vi "Outputs.vi"(8 "error in (no error)":errorcluster, 11 "State in":T1={"State"=enum."Idle", "Start Time"=timestamp(0 s since 1904-01-01), "Configuration"={"Cycle Period"=0.0, "PID 2 Parameters"={"Input Device"=enum."4-20mA", "Output Device"=enum."Default", "Setpoint"=0.0, "PID gains"={"proportional gain (Kc)"=0.0, "integral time (Ti, min)"=0.0, "derivative time (Td, min)"=100.0}, "output range"={"output low"=0.0, "output high"=1.0}}, "Manual Entry"=0.0, "Auto?"=TRUE, "4-20mA Input Settings"={"Input Channel "=0}, "4-20mA Out Settings"={"Output DAQ Task"=""}, "Input Channel Tag Name "=""}, "Current Time"=timestamp(0 s since 1904-01-01), "PID 1 Parameters"={"Setpoint"=0.0, "PID gains"={"proportional gain (Kc)"=1.0, "integral time (Ti, min)"=0.01, "derivative time (Td, min)"=0.0}}, "First Iteration"=FALSE, "Data"={"4-20mA Input"=0.0, "PID 2 Process Variable"=0.0, "PID 2 Output"=0.0, "4-20mA Output"=0.0}, "Process Name"="", "Pump On?"=enum."Off", "Input Error"=FALSE, "Output Error"=FALSE, "Log Started"=FALSE, "Current Setpoint"=0.0} {"Configuration"."PID 2 Parameters"."output range"."output low" format="%.2f"; "Configuration"."PID 2 Parameters"."output range"."output high" min=0.0 max=100.0 format="%.2f"; "Configuration"."PID 2 Parameters"."PID gains"."derivative time (Td, min)" format="%.3f"; "Configuration"."PID 2 Parameters"."PID gains"."integral time (Ti, min)" format="%.3f"; "Configuration"."PID 2 Parameters"."PID gains"."proportional gain (Kc)" format="%.3f"; "PID 1 Parameters"."PID gains"."derivative time (Td, min)" format="%.3f"; "PID 1 Parameters"."PID gains"."integral time (Ti, min)" format="%.3f"; "PID 1 Parameters"."PID gains"."proportional gain (Kc)" format="%.3f"}) -> (0 "error out":errorcluster, 3 "State out":T1={"State"=enum."Idle", "Start Time"=timestamp(0 s since 1904-01-01), "Configuration"={"Cycle Period"=0.0, "PID 2 Parameters"={"Input Device"=enum."4-20mA", "Output Device"=enum."Default", "Setpoint"=0.0, "PID gains"={"proportional gain (Kc)"=0.0, "integral time (Ti, min)"=0.0, "derivative time (Td, min)"=100.0}, "output range"={"output low"=0.0, "output high"=1.0}}, "Manual Entry"=0.0, "Auto?"=TRUE, "4-20mA Input Settings"={"Input Channel "=0}, "4-20mA Out Settings"={"Output DAQ Task"=""}, "Input Channel Tag Name "=""}, "Current Time"=timestamp(0 s since 1904-01-01), "PID 1 Parameters"={"Setpoint"=0.0, "PID gains"={"proportional gain (Kc)"=1.0, "integral time (Ti, min)"=0.01, "derivative time (Td, min)"=0.0}}, "First Iteration"=FALSE, "Data"={"4-20mA Input"=0.0, "PID 2 Process Variable"=0.0, "PID 2 Output"=0.0, "4-20mA Output"=0.0}, "Process Name"="", "Pump On?"=enum."Off", "Input Error"=FALSE, "Output Error"=FALSE, "Log Started"=FALSE, "Current Setpoint"=0.0} {"Configuration"."PID 2 Parameters"."output range"."output low" format="%.2f"; "Configuration"."PID 2 Parameters"."output range"."output high" min=0.0 max=100.0 format="%.2f"; "Configuration"."PID 2 Parameters"."PID gains"."derivative time (Td, min)" format="%.3f"; "Configuration"."PID 2 Parameters"."PID gains"."integral time (Ti, min)" format="%.3f"; "Configuration"."PID 2 Parameters"."PID gains"."proportional gain (Kc)" format="%.3f"; "PID 1 Parameters"."PID gains"."derivative time (Td, min)" format="%.3f"; "PID 1 Parameters"."PID gains"."integral time (Ti, min)" format="%.3f"; "PID 1 Parameters"."PID gains"."proportional gain (Kc)" format="%.3f"})   [LabVIEW 2018, in "4-20mA Module.lvlib" / "4-20mA Module Engine.lvlib"]
uses:
  4-20mA Module Engine.lvlib
  State Cluster.ctl
  State Enum.ctl
  Pressure Transmitter/Pressure Transmitter Device Settings.ctl
  Pressure Reg Module/Pressure Regulator Device Settings.ctl
  Measure Instrument/PID 1 Parameters Cluster.ctl
  Tag VIs/Tag FGV Operation Enum.ctl
  Shared Variables/Dynamic Shared Variables.lvlib
  Pressure Reg Module/Pressure Regulator Library.lvlib
  Flow Regulator/Pressure Reg Module/Flow Regulator Library.lvlib
  Pressure Transmitter/Pressure Transmitter Library.lvlib
panel:
  # "Instrument Settings"
  # "Instrument Settings"
  # "Instrument Settings"
  # "Instrument Settings"
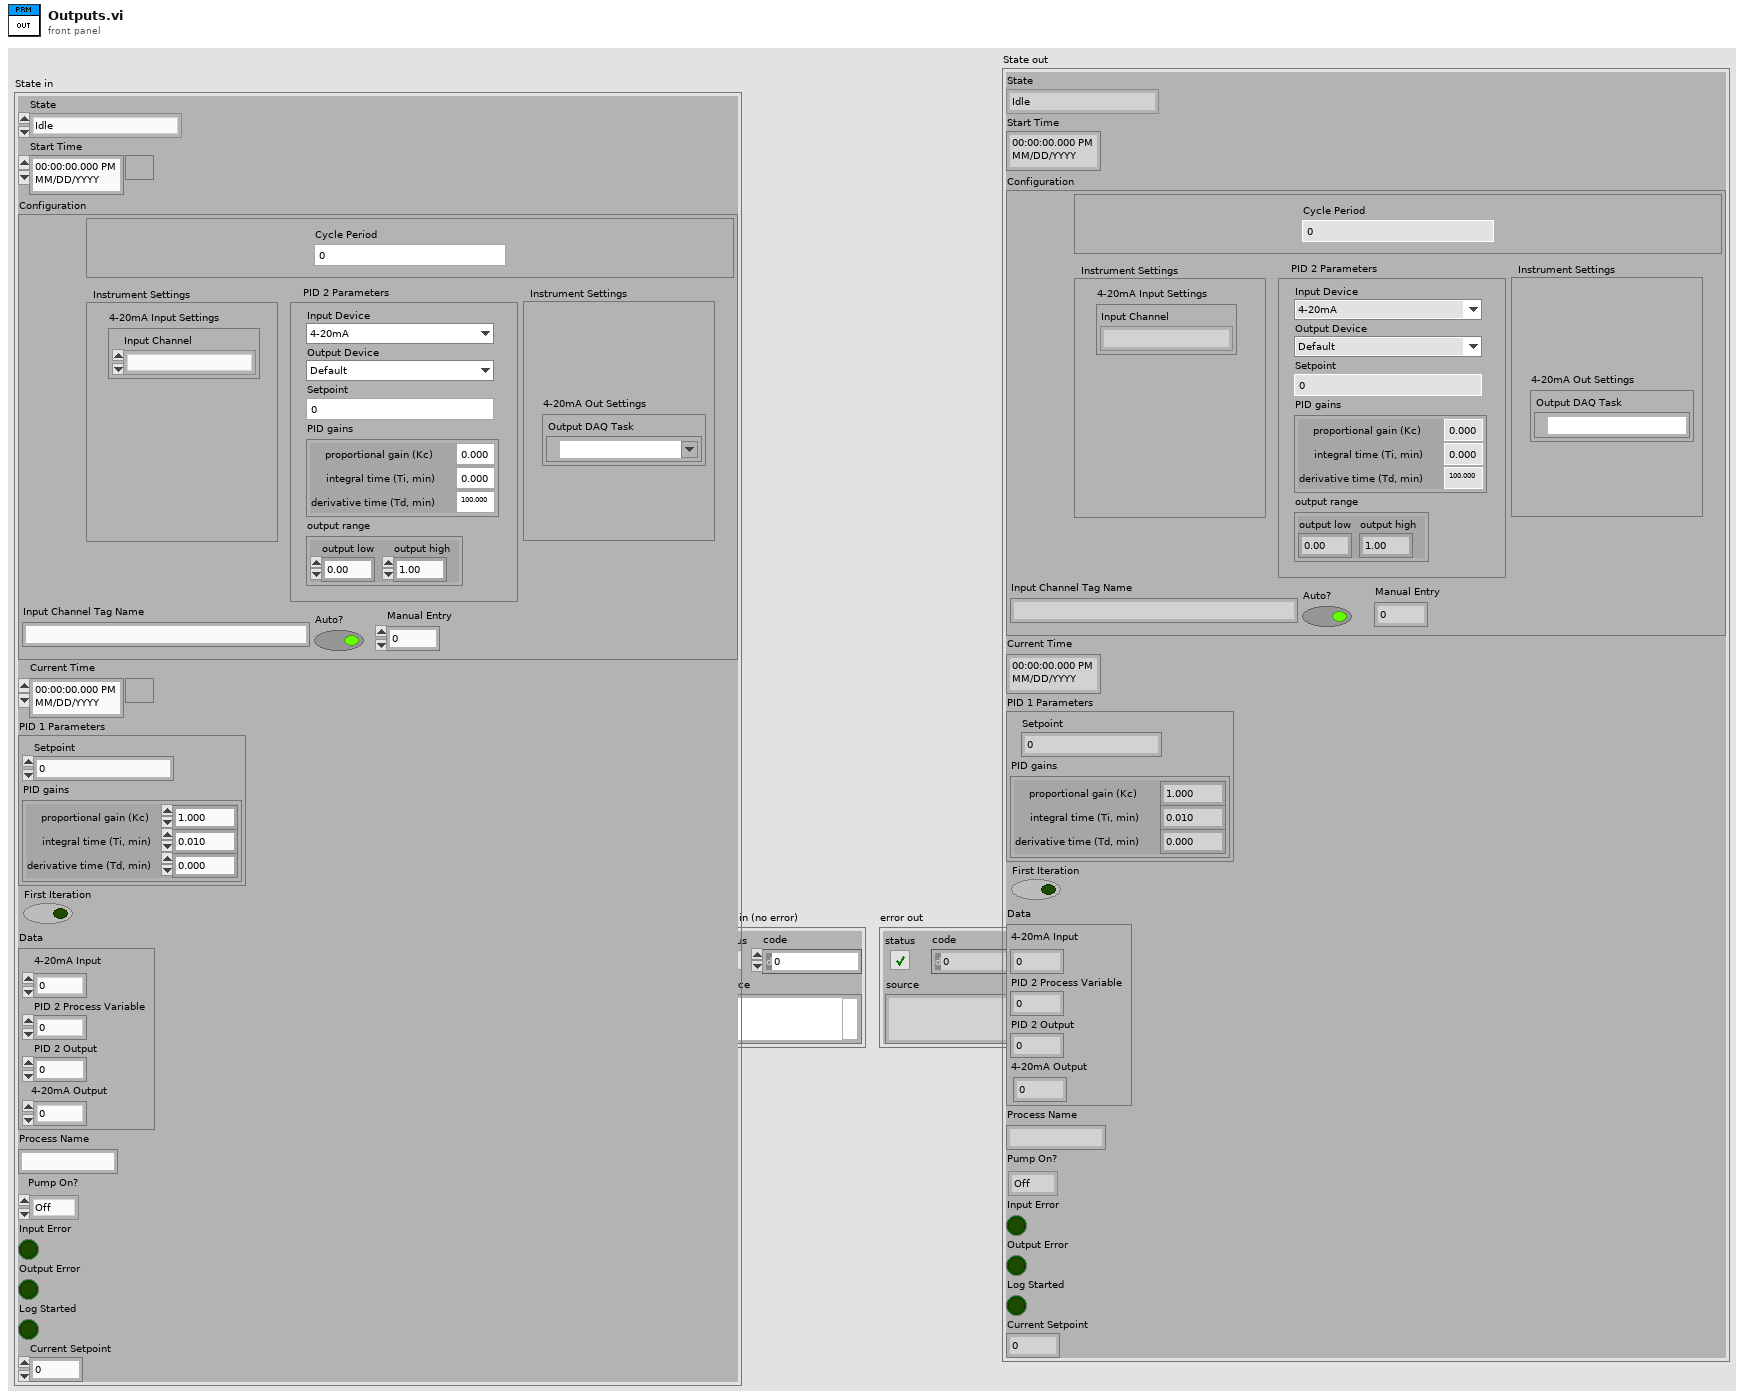
[diagram p1: front panel]
types:
  T1 = typedef "4-20mA Module.lvlib/4-20mA Module Engine.lvlib/State Cluster.ctl" = cluster{"State":T2, "Start Time":timestamp, "Configuration":cluster{"Cycle Period":dbl, "PID 2 Parameters":cluster{"Input Device":enum16{"Default", "4-20mA"}, "Output Device":enum16{"Default", "Equilibar Pressure Reg", "Flow Regulator"}, "Setpoint":dbl, "PID gains":cluster{"proportional gain (Kc)":dbl, "integral time (Ti, min)":dbl, "derivative time (Td, min)":dbl}, "output range":cluster{"output low":dbl, "output high":dbl}}, "Manual Entry":dbl, "Auto?":bool, "4-20mA Input Settings":T3, "4-20mA Out Settings":T4, "Input Channel Tag Name ":string}, "Current Time":timestamp, "PID 1 Parameters":T5, "First Iteration":bool, "Data":cluster{"4-20mA Input":dbl, "PID 2 Process Variable":dbl, "PID 2 Output":dbl, "4-20mA Output":dbl}, "Process Name":string, "Pump On?":enum16{"Off", "On", "Not Initialized"}, "Input Error":bool, "Output Error":bool, "Log Started":bool, "Current Setpoint":dbl}
  T2 = typedef "4-20mA Module.lvlib/4-20mA Module Engine.lvlib/State Enum.ctl" = enum16{"Measuring", "Idle", "Paused"}
  T3 = typedef "Pressure Transmitter Library.lvlib/Pressure Transmitter Device Settings.ctl" = cluster{"Input Channel ":u16}
  T4 = typedef "Pressure Regulator Library.lvlib/Pressure Regulator Device Settings.ctl" = cluster{"Output DAQ Task":refnum<k21>}
  T5 = typedef "PID 1 Parameters Cluster.ctl" = cluster{"Setpoint":dbl, "PID gains":cluster{"proportional gain (Kc)":dbl, "integral time (Ti, min)":dbl, "derivative time (Td, min)":dbl}}
  T6 = typedef "Tag FGV Operation Enum.ctl" = enum16{"Init", "Set Notification Queue", "Create Tag", "Commit", "Write Tag (Numeric)", "Write Tag (Boolean)", "Read All Tags", "Read One Tag", "Delete Tag Category", "Set Alarm Parameters (Numeric)", "Set Alarm Parameters (Boolean)", "Enable All Alarms", "Disable All Alarms", "Delete All Tags", "Read Alarms", "Ack Alarm", "Read Alarm Parameters (Numeric)", "Read Alarm Parameters (Boolean)"}
  T7 = enum16{"Default", "Equilibar Pressure Reg", "Flow Regulator"}
  T8 = typedef "4-20mA Module.lvlib/4-20mA Module Tag Names Cluster.ctl" = cluster{"4-20mA Input":string, "PID 2 Out Tag":string, "4-20mA Output":string, "Input Device Tag":string, "Output Device Tag":string}
  T9 = typedef "Flow Regulator Library.lvlib/Pressure Regulator Device Settings.ctl" = cluster{"Output DAQ Task":refnum<k21>}
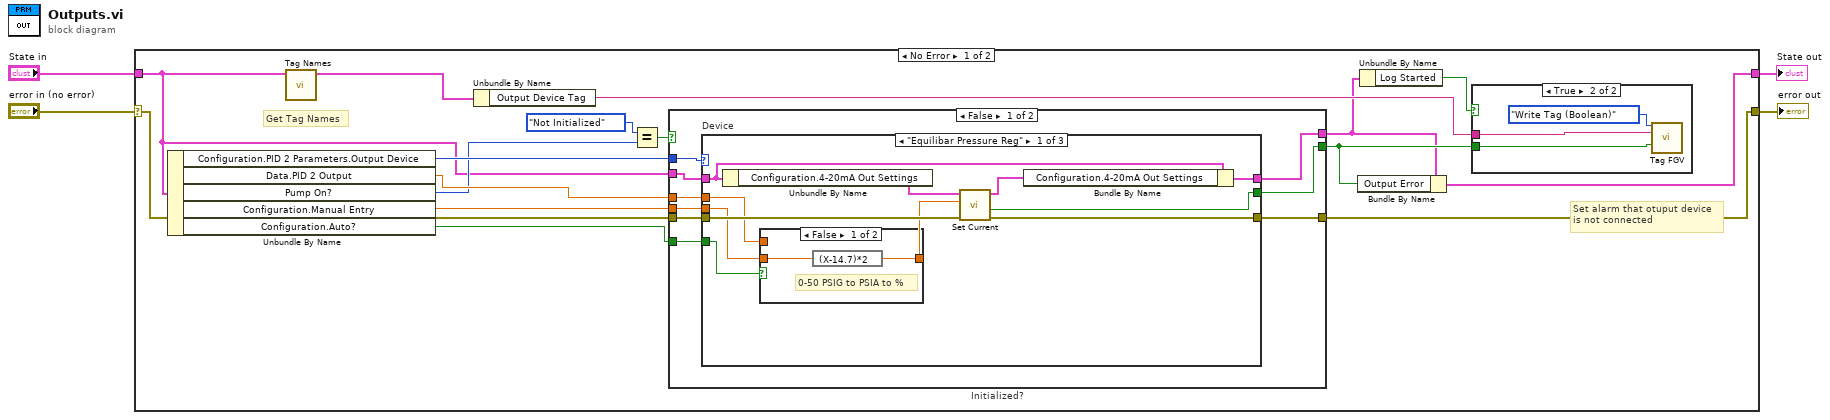
[diagram p0: block diagram]
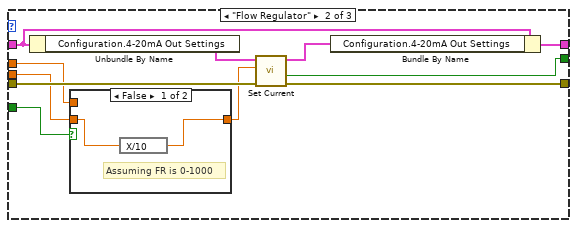
[diagram p4: hidden frame]
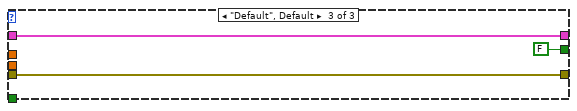
[diagram p6: hidden frame]
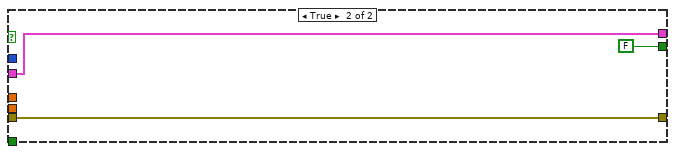
[diagram p7: hidden frame]
diagram:
  n1 = case shown="No Error" "error in (no error)" {
    selector: "error in (no error)" -> [w18 w68]
    tunnel: [w16 w68] -> w3
    tunnel: "State in" -> [w7 w67]
    tunnel: [w14 w67] -> w1
    frame No Error {
      # "Get Tag Names"
      # "Set alarm that otuput device\nis not connected"
      n2 = Unbundle By Name(w7) -> ("Configuration.PID 2 Parameters.Output Device"=w20:T7, "Data.PID 2 Output"=w19:dbl, "Pump On?"=w12:enum16{"Off", "On", "Not Initialized"}, "Configuration.Manual Entry"=w5:dbl, "Configuration.Auto?"=w6:bool)
      n3 = call "Tag Names.vi"("State in"=w7) -> ("4-20mA Module Tag Names"=w17:T8)  [unwired: 8 in, 2 out]
      n4 = Unbundle By Name(w17) -> ("Output Device Tag"=w15:string)
      n5 = Equal?(x=enum16{"Off", "On", "Not Initialized"}."Not Initialized", y=w12) -> (x = y?=w10:bool)
      n6 = case "Initialized?" shown="False" w10 {
        tunnel: w20 -> [w32 _]
        tunnel: w19 -> [w31 _]
        tunnel: w18 -> [w30 w65]
        tunnel: [w29 w65] -> w16
        tunnel: w7 -> [w28 w66]
        tunnel: [w27 w66] -> w9
        tunnel: [w26 FALSE ("Connection Error")] -> w13
        tunnel: w6 -> [w25 _]
        tunnel: w5 -> [w24 _]
        frame False {
          n7 = case "Device" shown="\"Equilibar Pressure Reg\"" w32 {
            tunnel: w31 -> [w36 w49 _]
            tunnel: w30 -> [w43 w54 w62]
            tunnel: [w42 w51 w62] -> w29
            tunnel: w28 -> [w41 w57 w63]
            tunnel: [w38 w56 w63] -> w27
            tunnel: [w37 w52 FALSE ("Connection Error")] -> w26
            tunnel: w25 -> [w33 w50 _]
            tunnel: w24 -> [w35 w47 _]
            frame "Equilibar Pressure Reg" {
              n8 = Unbundle By Name(w41) -> ("Configuration.4-20mA Out Settings"=w40:T4)
              n9 = case shown="False" w33 {
                tunnel: w36 -> [_ w46]
                tunnel: [w45 w46] -> w34
                tunnel: w35 -> [w44 _]
                frame False {
                  # "0-50 PSIG to PSIA to %"
                  n10 = expression code="(X-14.7)*2"(w44) -> (w45:dbl)
                }
                frame True {
                }
              }
              n11 = call "Set Current.vi"("error in"=w43, "%"=w34, "4-20mA Out Settings In"=w40) -> ("error out"=w42:errorcluster, "Connection Error"=w37:bool, "4-20mA Out Settings Out"=w39:T4)  [unwired: 6 in]
              n12 = Bundle By Name(cluster=w41, "Configuration.4-20mA Out Settings"=w39) -> (w38:T1)
            }
            frame "Flow Regulator" {
              n13 = Unbundle By Name(w57) -> ("Configuration.4-20mA Out Settings"=w55:T4)
              n14 = case shown="False" w50 {
                tunnel: w49 -> [_ w60]
                tunnel: [w59 w60] -> w48
                tunnel: w47 -> [w58 _]
                frame False {
                  # "Assuming FR is 0-1000"
                  n15 = expression code="X/10"(w58) -> (w59:dbl)
                }
                frame True {
                }
              }
              n16 = call "Set Current.vi"("error in"=w54, "%"=w48, "4-20mA Out Settings In"=w55) -> ("error out"=w51:errorcluster, "Connection Error"=w52:bool, "4-20mA Out Settings Out"=w53:T9)  [unwired: 6 in]
              n17 = Bundle By Name(cluster=w57, "Configuration.4-20mA Out Settings"=w53) -> (w56:T1)
            }
            frame "Default", Default {
            }
          }
        }
        frame True {
        }
      }
      n18 = Bundle By Name(cluster=w9, "Output Error"=w13) -> (w14:T1)
      n19 = Unbundle By Name(w9) -> ("Log Started"=w8:bool)
      n20 = case shown="True" w8 {
        tunnel: w15 -> [_ w23]
        tunnel: w13 -> [_ w21]
        frame False {
        }
        frame True {
          n21 = call "Tag FGV.vi"("Operation"=Tag_FGV_Operation_Enum."Write Tag (Boolean)", "Tag Name"=w23, "Data"=w21) -> ()  [unwired: 5 in, 8 out]
        }
      }
    }
    frame Error {
    }
  }
  "error out" <- w3
  "State out" <- w1
